vi "Enable Disable Add Remove buttons.vi"(5 "Force add disabled (F)":bool, 6 "reserved item indexes":i32[](array[numeric]), 7 "not present item indexes":i32[](array[numeric]), 8 "error in (no error)":errorcluster, 9 "selected items":i32[](array[numeric]), 10 "remove button":refnum<vi>, 11 "add button":refnum<vi>) -> (0 "error out":errorcluster)   [LabVIEW 2016, in "FPGA Addon System Explorer.lvlib"]
uses:
  FPGA Addon System Explorer.lvlib
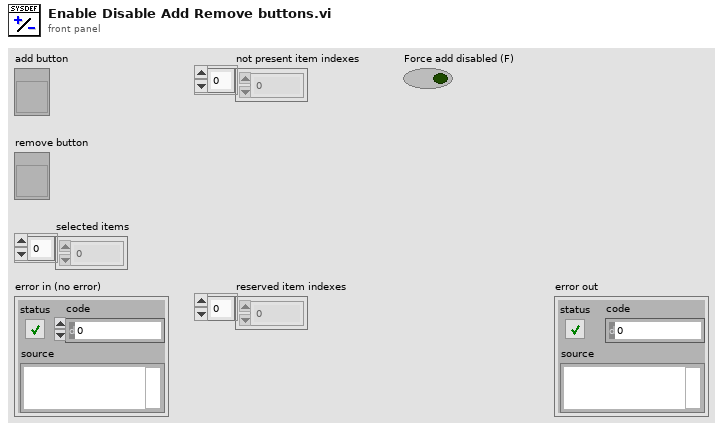
[diagram p1: front panel]
types:
  T1 = enum8{"Enabled", "Disabled", "Disabled and Grayed Out"}
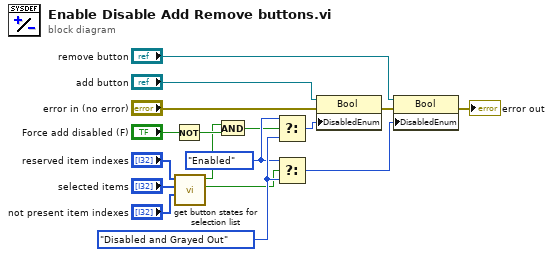
[diagram p0: block diagram]
diagram:
  w8 = T1."Disabled and Grayed Out" ("Disabled")
  w7 = T1."Enabled" ("Disabled")
  n1 = Not(x="Force add disabled (F)") -> (.not. x?=w3:bool)
  n2 = call "get button states for selection list.vi"("not present item indexes"="not present item indexes", "selected items"="selected items", "reserved item indexes"="reserved item indexes") -> ("remove enable"=w5:bool, "add enable"=w2:bool)  [unwired: 7 in]
  n3 = And(x=w2, y=w3) -> (x .and. y?=w1:bool)
  n4 = Select(t=w7, s=w1, f=w8) -> (s? t:f=w10:T1)
  n5 = Select(t=w7, s=w5, f=w8) -> (s? t:f=w9:T1)
  n6 = property on="Property Node" class="Bool"(reference="add button", error in="error in (no error)", "DisabledEnum"=w10) -> (error out=w15:errorcluster)  [unwired: 1 out]
  n7 = property on="Property Node" class="Bool"(reference="remove button", error in=w15, "DisabledEnum"=w9) -> (error out=→"error out":errorcluster)  [unwired: 1 out]
